vi "根据角度计算旋转程式序号.vi"(11 "角度(-90~90)":dbl) -> (1 "拧紧程式序号数组":i32[](array[numeric]), 2 "旋转程式序号 2":i32, 3 "旋转程式序号":i32)   [LabVIEW 2014]
panel:
  out "旋转角度2":i32
  out "旋转角度1":i32
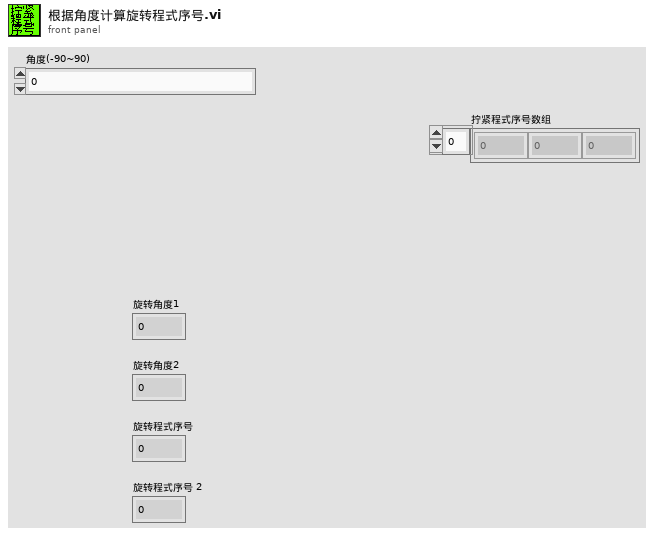
[diagram p1: front panel]
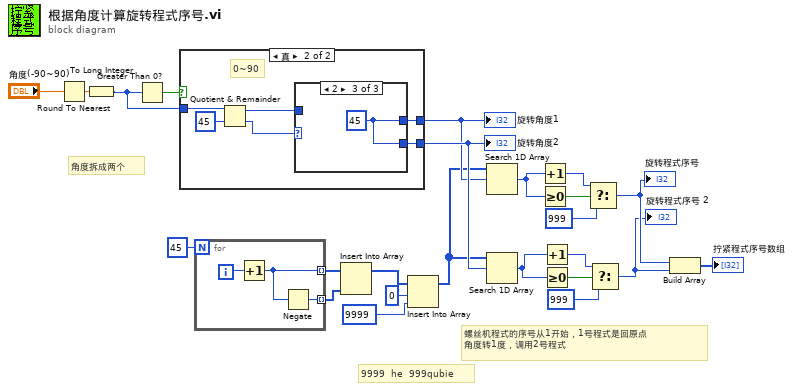
[diagram p0: block diagram]
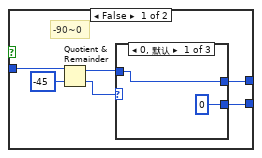
[diagram p2: hidden frame]
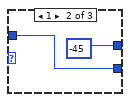
[diagram p3: hidden frame]
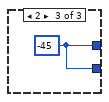
[diagram p4: hidden frame]
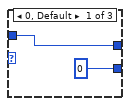
[diagram p5: hidden frame]
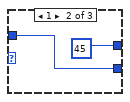
[diagram p6: hidden frame]
diagram:
  # "9999  he  999qubie"
  # "螺丝机程式的序号从1开始，1号程式是回原点\n角度转1度，调用2号程式"
  # "角度拆成两个"
  n1 = Round To Nearest(number="角度(-90~90)") -> (nearest integer value=w21:dbl)
  n2 = To Long Integer(number=w21) -> (32bit integer=w22:i32)
  n3 = Greater Than 0?(x=w22) -> (x > 0?=w16:bool)
  n4 = case shown="真" w16 {
    tunnel: w22 -> [w29 w41]
    tunnel: [w28 w39] -> w23
    tunnel: [w27 w37] -> w24
    frame False {
      # "-90~0"
      n5 = Quotient & Remainder(x=w29, y=-45) -> (x-y*floor(x/y)=w26:i32, floor(x/y)=w25:i32)
      n6 = case shown="0, 默认" w25 {
        tunnel: [w31 -45 ("f") w35] -> w28
        tunnel: w26 -> [w31 w34 _]
        tunnel: [0 ("t") w34 w35] -> w27
        frame 0, Default {
        }
        frame 1 {
        }
        frame 2 {
          w35 = -45 ("f")
        }
      }
    }
    frame True {
      # "0~90"
      n7 = Quotient & Remainder(x=w41, y=45) -> (x-y*floor(x/y)=w38:i32, floor(x/y)=w36:i32)
      n8 = case shown="2" w36 {
        tunnel: [w43 45 ("f") w46] -> w39
        tunnel: w38 -> [w43 w45 _]
        tunnel: [0 ("t") w45 w46] -> w37
        frame 0, Default {
        }
        frame 1 {
        }
        frame 2 {
          w46 = 45 ("f")
        }
      }
    }
  }
  "旋转角度1" <- w23
  "旋转角度2" <- w24
  n9 = for {
    N: 45 -> [_]
    tunnel: [w48] -> w18 mode=indexing
    tunnel: [w47] -> w19 mode=indexing
    i -> [w49]
    n10 = Increment(x=w49) -> (x+1=w48:i32)
    n11 = Negate(x=w48) -> (-x=w47:i32)
  }
  n12 = Insert Into Array(array=w18, new element=w19) -> (w4:i32[])  [unwired: 1 in]
  n13 = Insert Into Array(array=w4, index=0 ("索引"), new element=9999 ("新元素/子数组")) -> (w1:i32[])
  n14 = Search 1D Array(1D array=w1, element=w23) -> (index of element=w10:i32)  [unwired: 1 in]
  n15 = Search 1D Array(1D array=w1, element=w24) -> (index of element=w6:i32)  [unwired: 1 in]
  n16 = Increment(x=w10) -> (x+1=w13:i32)
  n17 = Greater Or Equal To 0?(x=w10) -> (x >= 0?=w14:bool)
  n18 = Increment(x=w6) -> (x+1=w8:i32)
  n19 = Greater Or Equal To 0?(x=w6) -> (x >= 0?=w7:bool)
  n20 = Select(t=w13, s=w14, f=999) -> (s? t:f=w11:i32)
  "旋转程式序号" <- w11
  n21 = Select(t=w8, s=w7, f=999) -> (s? t:f=w5:i32)
  "旋转程式序号 2" <- w5
  n22 = Build Array(w11, w5) -> (→"拧紧程式序号数组":i32[])
